vi "AddComment.vi"(7 "Time (Now)":timestamp, 8 "error in":errorcluster, 10 "Comment":string, 11 "Defect in":refnum<class "Defect.lvclass">) -> (0 "error out":errorcluster, 2 "Comment":refnum<class "UserComment.lvclass">, 3 "Defect out":refnum<class "Defect.lvclass">)   [LabVIEW 2021, in "ProligentXMLGenerator.lvlib" / "Defect.lvclass"]
doc: "Add a comment.\n\nRepresents a comment made by a user at a given time. Note that a user comment is considered unique when the comment, user and time are equal for a given associated fact. For example, if two failures have the same comment, user and time, they will be considered as two different comments because they are not attached to the same failure. But if two xmls are received by the DIT and they contain the same comment, user and time for the same failure ID, then they will be considered the same comment and the second comment will be discarded silently by the DIT."
uses:
  Defect.lvclass
  Defect.lvclass/Defect.ctl
  Model/UserComment/UserComment.lvclass
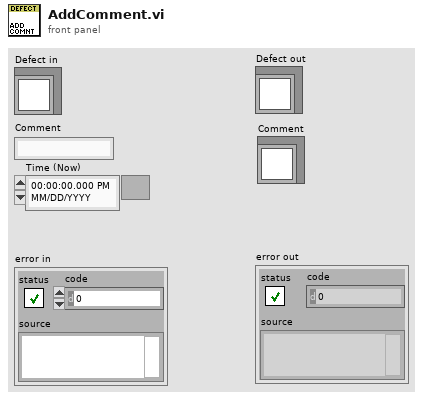
[diagram p1: front panel]
types:
  T1 = typedef "ProligentXMLGenerator.lvlib/Defect.lvclass/Data.ctl" = cluster{"Name":string, "Comments":refnum<class "UserComment.lvclass">[], "CustomData":refnum<class "CustomData.lvclass">, "DefectId":refnum<class "Guid.lvclass">, "OpenTime":refnum<class "DateTime.lvclass">, "TimeZoneInfoId":string}
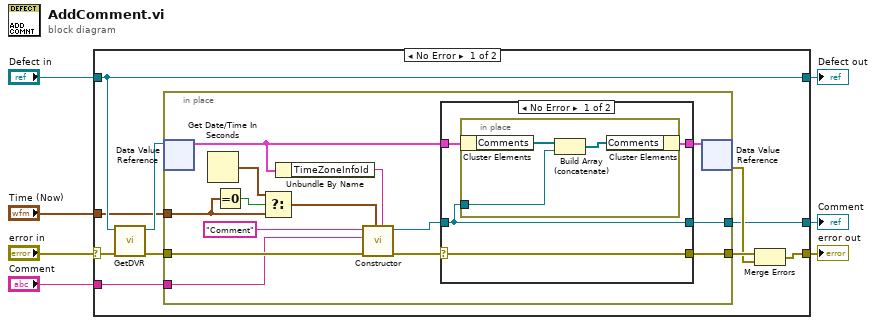
[diagram p0: block diagram]
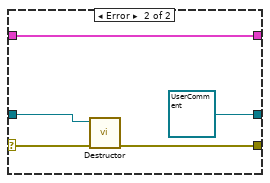
[diagram p2: hidden frame]
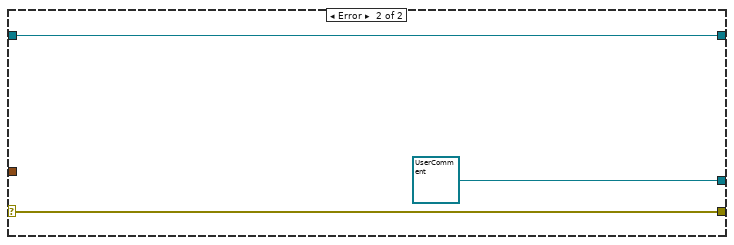
[diagram p3: hidden frame]
diagram:
  n1 = case shown="No Error" "error in" {
    selector: "error in" -> [w15 w46]
    tunnel: [w11 w46] -> w7
    tunnel: [w12 w45] -> w5
    tunnel: "Defect in" -> [w12 w45]
    tunnel: "Comment" -> [w17 _]
    tunnel: [w9 refnum<class "UserComment.lvclass"> refnum ("UserComment out")] -> w2
    tunnel: "Time (Now)" -> [w8 _]
    frame No Error {
      n2 = call "GetDVR.vi"("error in"=w15, "Defect"=w12) -> ("error out"=w14:errorcluster, "DVRReference"=w13:refnum<data-value>)  [unwired: 8 in]
      n3 = in-place "In Place Element Structure" {
        in-place-border: w17 -> [w24]
        in-place-border: [w30] -> w16
        in-place-border: w14 -> [w29]
        in-place-border: [w27] -> w9
        in-place-border: w8 -> [w21]
        n4 = in-place-dvr #1(w13) -> (w19:T1)  [unwired: 1 out]
        n5 = Get Date/Time In Seconds() -> (seconds since 1Jan1904=w22:timestamp)
        n6 = Equal To 0?(x=w21) -> (x = 0?=w23:bool)
        n7 = Select(t=w22, s=w23, f=w21) -> (s? t:f=w20:timestamp)
        n8 = Unbundle By Name(w19) -> ("TimeZoneInfoId"=w18:string)
        n9 = call "Constructor.vi"("TimeZoneInfoId"=w18, "Time"=w20, "error in"=w29, "Comment"=w24, "Name"="Comment") -> ("error out"=w31:errorcluster, "UserComment out"=w26:refnum<class "UserComment.lvclass">)  [unwired: 5 in]
        n10 = case shown="No Error" w31 {
          selector: w31 -> [w35 w41]
          tunnel: [w32 w43] -> w28
          tunnel: [w35 w40] -> w30
          tunnel: w26 -> [w34 w42]
          tunnel: w19 -> [w33 w43]
          tunnel: [w34 refnum<class "UserComment.lvclass"> refnum ("UserComment in")] -> w27
          frame No Error {
            n11 = in-place "In Place Element Structure" {
              in-place-border: w34 -> [w38]
              n12 = in-place-cluster #2(w33) -> ("Comments"=w37:refnum<class "UserComment.lvclass">[])
              n13 = Build Array (concatenate)(w37, w38) -> (w36:refnum<class "UserComment.lvclass">[])
              n14 = in-place-cluster #2("Comments"=w36) -> (w32:T1)
            }
          }
          frame Error {
            n15 = call "Destructor.vi"("error in"=w41, "UserComment"=w42) -> ("error out"=w40:errorcluster)  [unwired: 9 in]
          }
        }
        n16 = in-place-dvr #1(w28) -> (w10:errorcluster)  [unwired: 1 out]
      }
      n17 = Merge Errors(w16, w10) -> (w11:errorcluster)
    }
    frame Error {
    }
  }
  "error out" <- w7
  "Defect out" <- w5
  "Comment" <- w2
